vi "Write AxisNumber.vi"(8 "error in (no error)":errorcluster, 10 "AxisNumber":u8, 11 "ReferenceMove Msg in":refnum<class "ReferenceMove Msg.lvclass">) -> (0 "error out":errorcluster, 3 "ReferenceMove Msg out":refnum<class "ReferenceMove Msg.lvclass">)   [LabVIEW 2016, in "CS++Motor.lvlib" / "ReferenceMove Msg.lvclass"]
uses:
  ReferenceMove Msg.lvclass
  ReferenceMove Msg.lvclass/ReferenceMove Msg.ctl
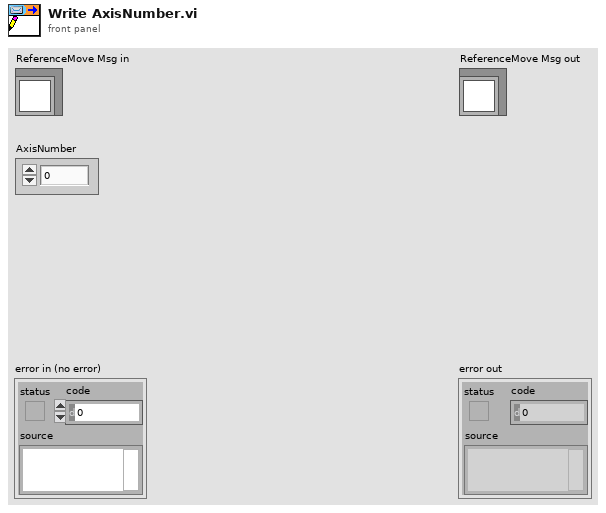
[diagram p1: front panel]
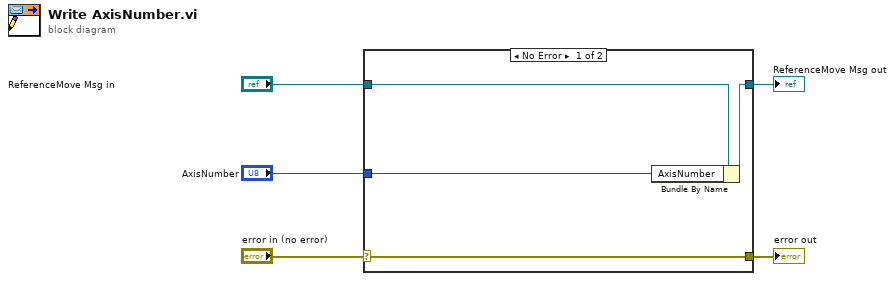
[diagram p0: block diagram]
diagram:
  n1 = case shown="No Error" "error in (no error)" {
    selector: "error in (no error)" -> [w9 w10]
    tunnel: [w9 w10] -> w4
    tunnel: [w7 w11] -> w2
    tunnel: "ReferenceMove Msg in" -> [w8 w11]
    tunnel: "AxisNumber" -> [w6 _]
    frame No Error {
      n2 = Bundle By Name(cluster=w8, "AxisNumber"=w6) -> (w7:refnum<class "ReferenceMove Msg.lvclass">)
    }
    frame Error {
    }
  }
  "error out" <- w4
  "ReferenceMove Msg out" <- w2
